vi "zuege (SubVI).vi"(11 "X Zug":bool) -> (2 "Boolesch":bool, 3 "Numerisch":i32)   [LabVIEW 2017]
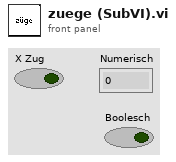
[diagram p1: front panel]
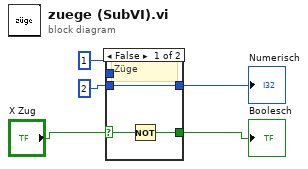
[diagram p0: block diagram]
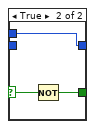
[diagram p2: hidden frame]
diagram:
  n1 = case shown="False" "X Zug" {
    selector: "X Zug" -> [w8 w11]
    tunnel: 1 -> [_ w9]
    tunnel: 2 -> [w6 _]
    tunnel: [w6 w9] -> w3
    tunnel: [w7 w10] -> w5
    frame False {
      # "Züge"
      n2 = Not(x=w8) -> (.not. x?=w7:bool)
    }
    frame True {
      n3 = Not(x=w11) -> (.not. x?=w10:bool)
    }
  }
  "Boolesch" <- w5
  "Numerisch" <- w3
